vi "LHPulse_ECD.vi"(1 "LHPulse(us)":T1, 2 "LHHeizen2?":T2, 3 "LHHeizen1?":T2) -> ()   [LabVIEW 2017]
uses:
  <vilib>/rvi/eio/common/nirviEmuTemplateMethod_errors.vi
  <vilib>/eio/EIONode/EIONode.xnode
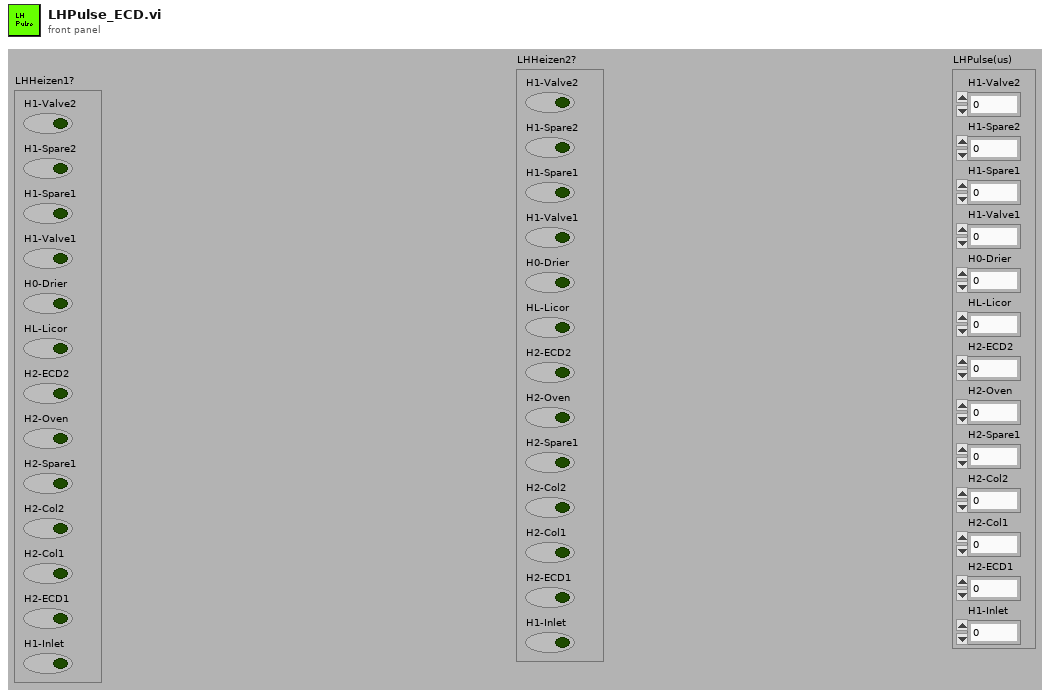
[diagram p1: front panel]
types:
  T1 = cluster{"H1-Valve2":u32, "H1-Spare2":u32, "H1-Spare1":u32, "H1-Valve1":u32, "H0-Drier":u32, "HL-Licor":u32, "H2-ECD2":u32, "H2-Oven":u32, "H2-Spare1":u32, "H2-Col2":u32, "H2-Col1":u32, "H2-ECD1":u32, "H1-Inlet":u32}
  T2 = cluster{"H1-Valve2":bool, "H1-Spare2":bool, "H1-Spare1":bool, "H1-Valve1":bool, "H0-Drier":bool, "HL-Licor":bool, "H2-ECD2":bool, "H2-Oven":bool, "H2-Spare1":bool, "H2-Col2":bool, "H2-Col1":bool, "H2-ECD1":bool, "H1-Inlet":bool}
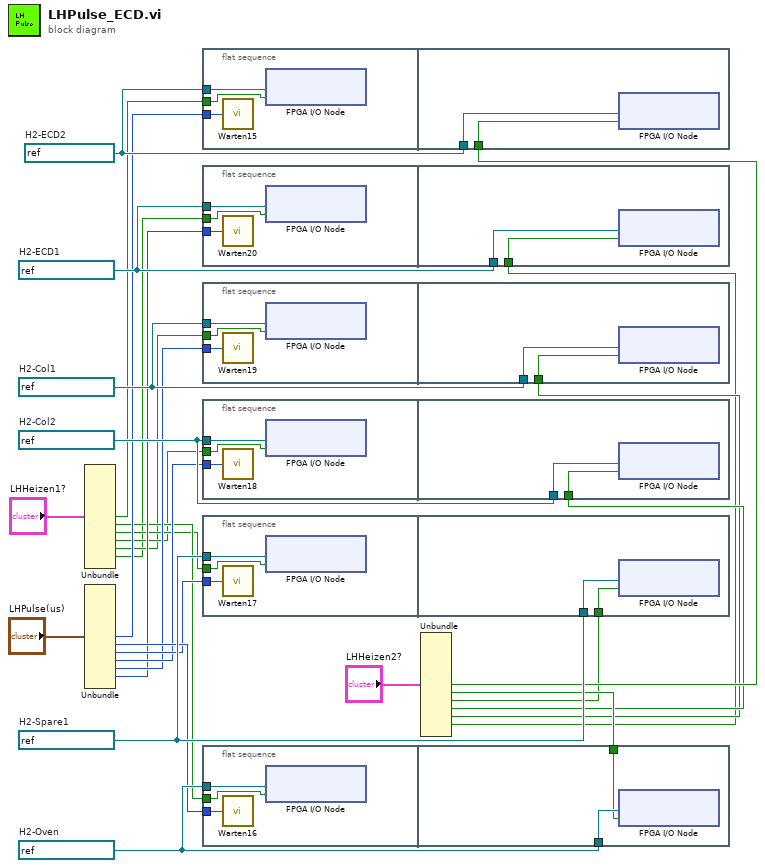
[diagram p0: block diagram]
diagram:
  w22 = refnum<k21> "Mod5/DIO20"  # H2-ECD1
  w23 = refnum<k21> "Mod5/DIO19"  # H2-Col1
  w24 = refnum<k21> "Mod5/DIO18"  # H2-Col2
  w25 = refnum<k21> "Mod5/DIO17"  # H2-Spare1
  w26 = refnum<k21> "Mod5/DIO16"  # H2-Oven
  w27 = refnum<k21> "Mod5/DIO1"  # H2-ECD2
  n1 = Unbundle("LHHeizen1?") -> ("H2-ECD2"=w15:bool, "H2-Oven"=w14:bool, "H2-Spare1"=w13:bool, "H2-Col2"=w12:bool, "H2-Col1"=w11:bool, "H2-ECD1"=w10:bool)  [unwired: 7 out]
  n2 = Unbundle("LHPulse(us)") -> ("H2-ECD2"=w21:u32, "H2-Oven"=w20:u32, "H2-Spare1"=w19:u32, "H2-Col2"=w18:u32, "H2-Col1"=w17:u32, "H2-ECD1"=w16:u32)  [unwired: 7 out]
  n3 = flat-sequence {
    tunnel: w27 -> [w30]
    tunnel: w15 -> [w29]
    tunnel: w21 -> [w28]
    tunnel: w27 -> [w32]
    tunnel: w9 -> [w31]
    frame #0 {
      n4 = call "Warten15"("Count(uSec)"=w28) -> ()  [unwired: 1 out]
      n5 = xnode "FPGA I/O Node"("I/O-Objekt"=w29, "FPGA-I/O (Eingang)"=w30) -> ()  [unwired: 1 out]
    }
    frame #1 {
      n6 = xnode "FPGA I/O Node"("I/O-Objekt"=w31, "FPGA-I/O (Eingang)"=w32) -> ()  [unwired: 1 out]
    }
  }
  n7 = flat-sequence {
    tunnel: w22 -> [w35]
    tunnel: w10 -> [w34]
    tunnel: w16 -> [w33]
    tunnel: w22 -> [w37]
    tunnel: w4 -> [w36]
    frame #0 {
      n8 = call "Warten20"("Count(uSec)"=w33) -> ()  [unwired: 1 out]
      n9 = xnode "FPGA I/O Node"("I/O-Objekt"=w34, "FPGA-I/O (Eingang)"=w35) -> ()  [unwired: 1 out]
    }
    frame #1 {
      n10 = xnode "FPGA I/O Node"("I/O-Objekt"=w36, "FPGA-I/O (Eingang)"=w37) -> ()  [unwired: 1 out]
    }
  }
  n11 = flat-sequence {
    tunnel: w23 -> [w40]
    tunnel: w11 -> [w39]
    tunnel: w17 -> [w38]
    tunnel: w23 -> [w42]
    tunnel: w5 -> [w41]
    frame #0 {
      n12 = call "Warten19"("Count(uSec)"=w38) -> ()  [unwired: 1 out]
      n13 = xnode "FPGA I/O Node"("I/O-Objekt"=w39, "FPGA-I/O (Eingang)"=w40) -> ()  [unwired: 1 out]
    }
    frame #1 {
      n14 = xnode "FPGA I/O Node"("I/O-Objekt"=w41, "FPGA-I/O (Eingang)"=w42) -> ()  [unwired: 1 out]
    }
  }
  n15 = flat-sequence {
    tunnel: w24 -> [w45]
    tunnel: w12 -> [w44]
    tunnel: w18 -> [w43]
    tunnel: w24 -> [w47]
    tunnel: w6 -> [w46]
    frame #0 {
      n16 = call "Warten18"("Count(uSec)"=w43) -> ()  [unwired: 1 out]
      n17 = xnode "FPGA I/O Node"("I/O-Objekt"=w44, "FPGA-I/O (Eingang)"=w45) -> ()  [unwired: 1 out]
    }
    frame #1 {
      n18 = xnode "FPGA I/O Node"("I/O-Objekt"=w46, "FPGA-I/O (Eingang)"=w47) -> ()  [unwired: 1 out]
    }
  }
  n19 = flat-sequence {
    tunnel: w25 -> [w50]
    tunnel: w13 -> [w49]
    tunnel: w19 -> [w48]
    tunnel: w25 -> [w52]
    tunnel: w7 -> [w51]
    frame #0 {
      n20 = call "Warten17"("Count(uSec)"=w48) -> ()  [unwired: 1 out]
      n21 = xnode "FPGA I/O Node"("I/O-Objekt"=w49, "FPGA-I/O (Eingang)"=w50) -> ()  [unwired: 1 out]
    }
    frame #1 {
      n22 = xnode "FPGA I/O Node"("I/O-Objekt"=w51, "FPGA-I/O (Eingang)"=w52) -> ()  [unwired: 1 out]
    }
  }
  n23 = flat-sequence {
    tunnel: w26 -> [w55]
    tunnel: w14 -> [w54]
    tunnel: w20 -> [w53]
    tunnel: w26 -> [w57]
    tunnel: w8 -> [w56]
    frame #0 {
      n24 = call "Warten16"("Count(uSec)"=w53) -> ()  [unwired: 1 out]
      n25 = xnode "FPGA I/O Node"("I/O-Objekt"=w54, "FPGA-I/O (Eingang)"=w55) -> ()  [unwired: 1 out]
    }
    frame #1 {
      n26 = xnode "FPGA I/O Node"("I/O-Objekt"=w56, "FPGA-I/O (Eingang)"=w57) -> ()  [unwired: 1 out]
    }
  }
  n27 = Unbundle("LHHeizen2?") -> ("H2-ECD2"=w9:bool, "H2-Oven"=w8:bool, "H2-Spare1"=w7:bool, "H2-Col2"=w6:bool, "H2-Col1"=w5:bool, "H2-ECD1"=w4:bool)  [unwired: 7 out]
